vi "processUseControlBodyOnlyFlag_start.vi"(7 "useControlBodyOnly":bool, 8 "error in (no error)":errorcluster, 11 "refList":refnum<vi>[](array[refnum])) -> (0 "error out":errorcluster, 3 "refList(dup)":refnum<vi>[](array[refnum]), 4 "LabelVisibilityList":bool[](array[boolean]), 6 "captionVisibilityList":bool[](array[boolean]))   [LabVIEW 2023]
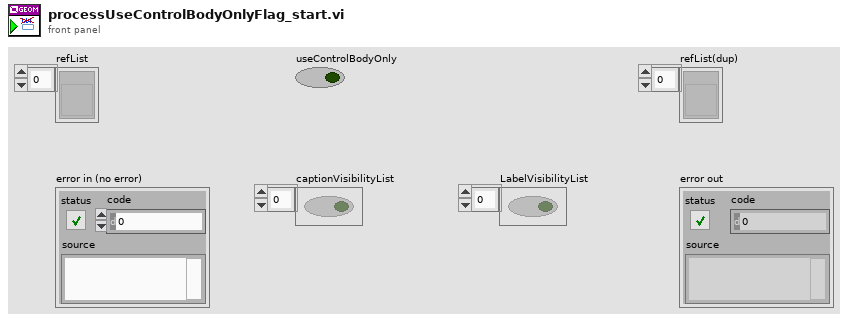
[diagram p1: front panel]
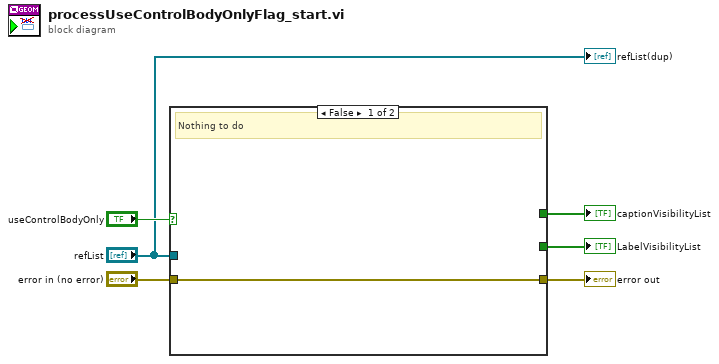
[diagram p0: block diagram]
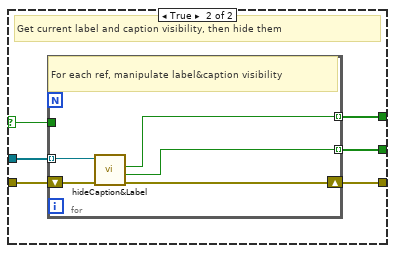
[diagram p2: hidden frame]
diagram:
  n1 = case shown="False" "useControlBodyOnly" {
    selector: "useControlBodyOnly" -> [_ w11]
    tunnel: "error in (no error)" -> [w7 w13]
    tunnel: [w7 w12] -> w5
    tunnel: "refList" -> [_ w10]
    tunnel: [_ w9] -> w2
    tunnel: [_ w8] -> w1
    frame False {
      # "Nothing to do"
    }
    frame True {
      # "Get current label and caption visibility, then hide them"
      n2 = for {
        tunnel: w10 -> [w16] mode=indexing
        shift-right: [w17] -> w12
        shift-left: w13 -> [w18]
        tunnel: w11 -> [_]
        tunnel: [w15] -> w9 mode=indexing
        tunnel: [w14] -> w8 mode=indexing
        # "For each ref, manipulate label&caption visibility"
        n3 = call "hideCaption&Label.vi"("error in (no error)"=w18, "Control in"=w16) -> ("error out"=w17:errorcluster, "Label.Visible"=w15:bool, "Caption.Visible"=w14:bool)  [unwired: 6 in, 1 out]
      }
    }
  }
  "LabelVisibilityList" <- w2
  "captionVisibilityList" <- w1
  "error out" <- w5
  "refList(dup)" <- "refList"
